vi "Check Absolute Time.vi"(8 "error in (no error)":errorcluster, 9 "Channel Name":string="Absolute Time", 10 "Group Name":string, 11 "Refnum in":refnum<k34>) -> (0 "error out":errorcluster, 1 "Last Absolute Time":dbl, 2 "Passed ?":bool, 3 "Refnum out":refnum<k34>)   [LabVIEW 2026, in "Telemetry System Tests.lvclass"]
uses:
  Telemetry System Tests.lvclass
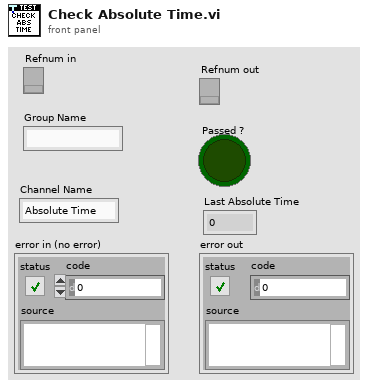
[diagram p1: front panel]
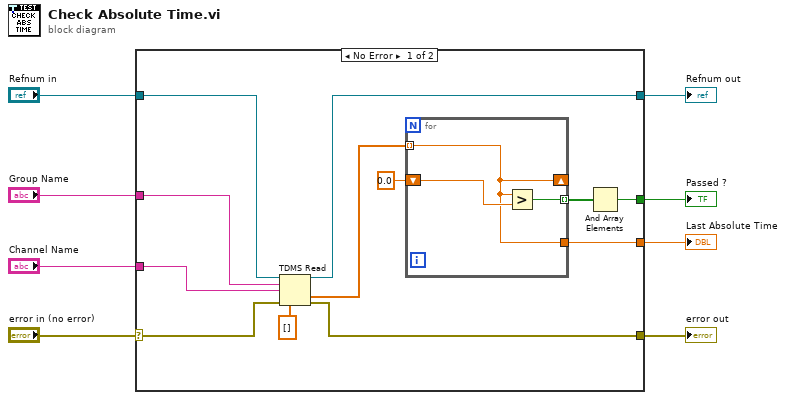
[diagram p0: block diagram]
diagram:
  n1 = case shown="No Error" "error in (no error)" {
    selector: "error in (no error)" -> [w17 w24]
    tunnel: [w20 w25] -> w8
    tunnel: [w12 w24] -> w7
    tunnel: "Refnum in" -> [w18 w25]
    tunnel: [w13 _] -> w4
    tunnel: [w11 _] -> w3
    tunnel: "Channel Name" -> [w10 _]
    tunnel: "Group Name" -> [w9 _]
    frame No Error {
      n2 = TDMS Read(0:w18, 5:w9, 7:w10, 11:w17, 12:dbl[] []) -> (4:w20:refnum<k34>, 10:w16:dbl[], 15:w12:errorcluster)  [unwired: 3 in, 3 out]
      n3 = for {
        tunnel: w16 -> [w21] mode=indexing
        shift-right: [w21] -> _
        shift-left: 0.0 -> [w23]
        tunnel: [w22] -> w14 mode=indexing
        tunnel: [w21] -> w11
        n4 = Greater?(x=w21, y=w23) -> (0:w22:bool)
      }
      n5 = And Array Elements(Boolean array=w14) -> (logical AND=w13:bool)
    }
    frame Error {
    }
  }
  "Refnum out" <- w8
  "error out" <- w7
  "Passed ?" <- w4
  "Last Absolute Time" <- w3
